vi "HMI.vi"() -> ()   [LabVIEW 2023]
uses:
  <vilib>/Instr/_visa.llb/VISA Configure Serial Port (Instr).vi
panel:
  out "reactiva":dbl
  out "aparente":dbl
  out "voltage":dbl
  out "corriente":dbl
  out "Fp":dbl
  in  "VISA resource name":refnum<visa-resource-name>
  out "Meter":dbl(knob) scale=0.001..1.0
  out "Voltaje (Señal control)":dynamicdata(graph)
  out "Numeric 3":dbl format="%#.2g"
  out "s? t:f 3":string
  out "s? t:f 2":string
  out "Numeric 2":dbl format="%#.2g"
  out "s? t:f":string
  out "Numeric":dbl format="%#.2g"
  in  "stop":bool
  out "1w 2":dbl(knob) scale=0.0..1.0
  out "10w 2":dbl(knob) scale=0.0..10.0
  out "100w":dbl(knob) scale=0.0..400.0
  out "10A 2":dbl(knob) scale=0.0..10.0
  out "1A":dbl(knob) scale=0.0..1.0
  out "1v":dbl(knob) scale=0.0..1.0
  out "10v":dbl(knob) scale=0.0..10.0
  out "100v":dbl(knob) scale=0.0..120.0
  # "ANALISIS ELECTRICO DEL SISTEMA ENERGETICO"
  # "Factor de Potencia"
  # "POTENCIA"
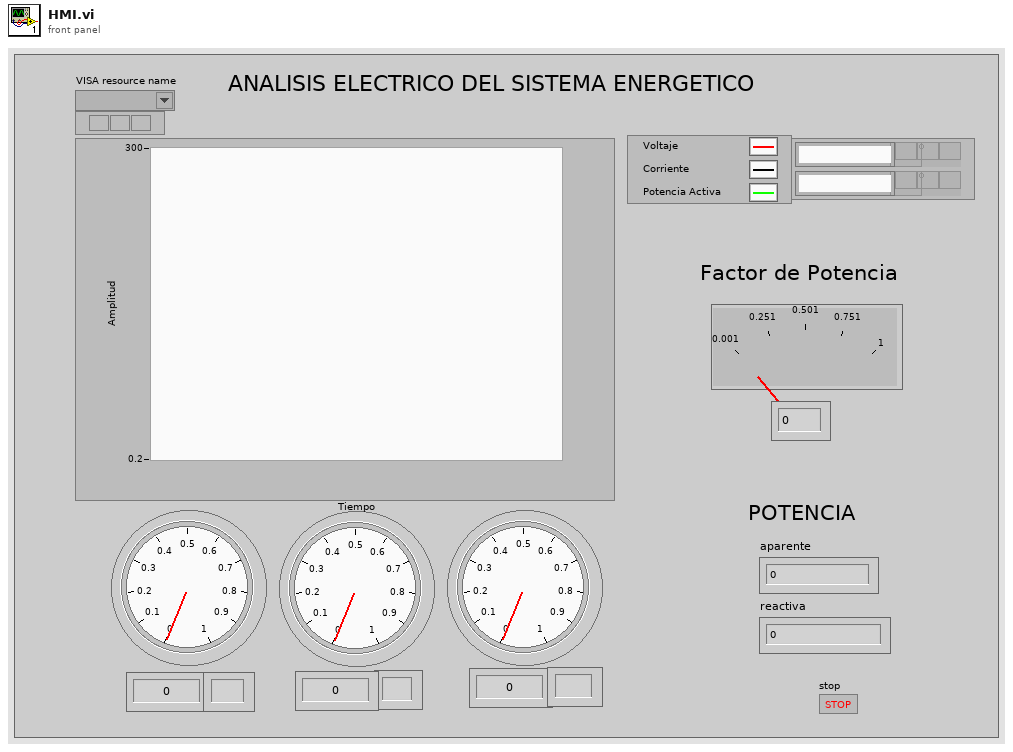
[diagram p1: front panel]
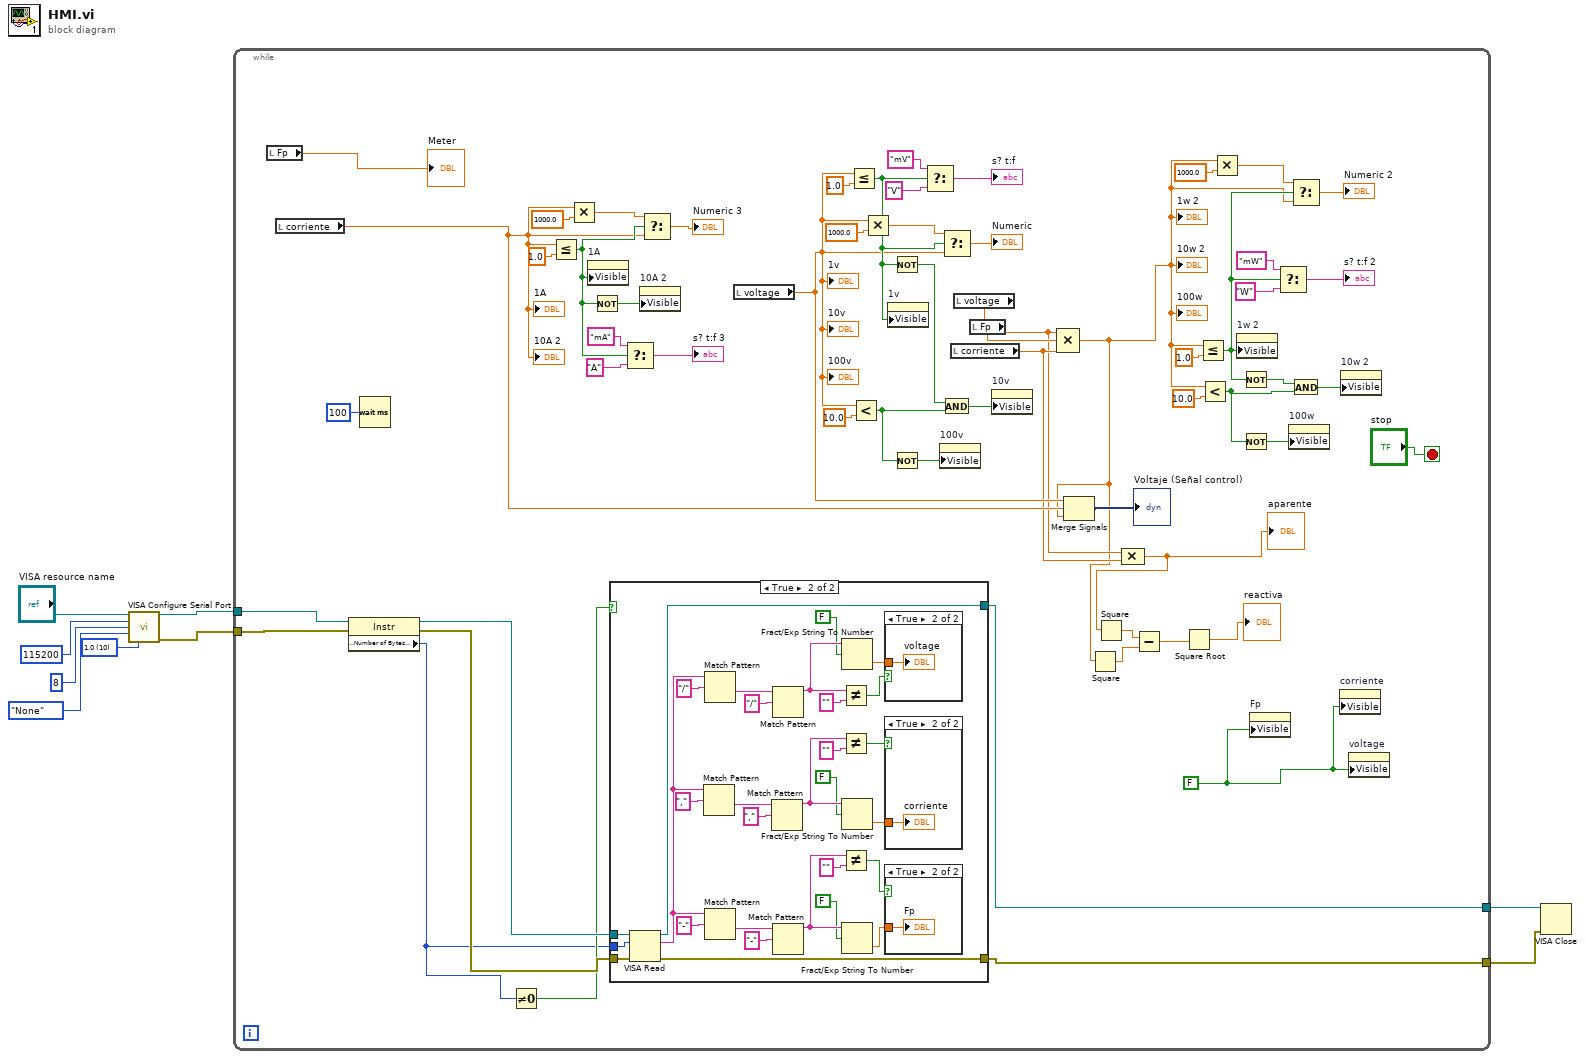
[diagram p0: block diagram]
diagram:
  w5 = u16 10 items=["1.0"=10, "1.5"=15, "2.0"=20] ("stop bits (10: 1 bit)")
  n1 = call-poly "VISA Configure Serial Port"("VISA resource name"="VISA resource name", "baud rate (9600)"=u32 115200, "data bits (8)"=u16 8, "parity (0:none)"=enum16{"None", "Odd", "Even", "Mark", "Space"}."None", "stop bits (10: 1 bit)"=w5) -> ("VISA resource name out"=w4:refnum<visa-resource-name>, "error out"=w3:errorcluster)  [unwired: 9 in]
  n2 = while {
    tunnel: w4 -> [w31]
    tunnel: w3 -> [w30]
    tunnel: [w26] -> w2
    tunnel: [w25] -> w1
    stop <- "stop" stop-if-true
    w22 = FALSE ("Visible")
    n3 = local read "Fp"() -> (→"Meter":dbl)
    n4 = local read "corriente"() -> (w20:dbl)
    "1A" <- w20
    "10A 2" <- w20
    n5 = property class="Instr"(reference=w31, error in=w30) -> (reference out=w28:refnum<visa-resource-name>, error out=w29:errorcluster, "Serial Settings:Number of Bytes at Serial Port"=w23:u32)
    n6 = Wait (ms)(milliseconds to wait=u32 100) -> ()  [unwired: 1 out]
    n7 = Not Equal To 0?(x=w23) -> (x != 0?=w24:bool)
    n8 = Less Or Equal?(x=w20, y=1.0) -> (x <= y?=w35:bool)
    n9 = Multiply(x=w20, y=1000.0) -> (x*y=w34:dbl)
    n10 = property on="1A" class="Knob (strict)"("Visible"=w35) -> ()  [unwired: 2 in, 2 out]
    n11 = Not(x=w35) -> (.not. x?=w38:bool)
    n12 = case shown="True" w24 {
      tunnel: [w69 w100] -> w25
      tunnel: [w70 w99] -> w26
      tunnel: w28 -> [w70 w98]
      tunnel: w29 -> [w69 w97]
      tunnel: w23 -> [_ w96]
      frame False {
      }
      frame True {
        n13 = VISA Read(VISA resource name=w98, byte count=w96, error in (no error)=w97) -> (VISA resource name out=w99:refnum<visa-resource-name>, read buffer=w86:string, error out=w100:errorcluster)  [unwired: 1 out]
        n14 = Match Pattern(string=w86, regular expression=",") -> (after substring=w93:string)  [unwired: 1 in, 3 out]
        n15 = Match Pattern(string=w86, regular expression="/") -> (after substring=w87:string)  [unwired: 1 in, 3 out]
        n16 = Match Pattern(string=w86, regular expression="-") -> (after substring=w90:string)  [unwired: 1 in, 3 out]
        n17 = Match Pattern(string=w93, regular expression=",") -> (before substring=w75:string)  [unwired: 1 in, 3 out]
        n18 = Match Pattern(string=w87, regular expression="/") -> (before substring=w84:string)  [unwired: 1 in, 3 out]
        n19 = Match Pattern(string=w90, regular expression="-") -> (before substring=w74:string)  [unwired: 1 in, 3 out]
        n20 = Not Equal?(x=w84, y="") -> (x != y?=w77:bool)
        n21 = Not Equal?(x=w75, y="") -> (x != y?=w79:bool)
        n22 = Not Equal?(x=w74, y="") -> (x != y?=w80:bool)
        n23 = Fract/Exp String To Number(use system decimal point (T)=FALSE, string=w84) -> (number=w76:dbl)  [unwired: 2 in, 1 out]
        n24 = Fract/Exp String To Number(use system decimal point (T)=FALSE, string=w75) -> (number=w78:dbl)  [unwired: 2 in, 1 out]
        n25 = Fract/Exp String To Number(use system decimal point (T)=FALSE, string=w74) -> (number=w81:dbl)  [unwired: 2 in, 1 out]
        n26 = case shown="True" w77 {
          tunnel: w76 -> [_ w103]
          frame False {
          }
          frame True {
            "voltage" <- w103
          }
        }
        n27 = case shown="True" w79 {
          tunnel: w78 -> [_ w102]
          frame False {
          }
          frame True {
            "corriente" <- w102
          }
        }
        n28 = case shown="True" w80 {
          tunnel: w81 -> [_ w101]
          frame False {
          }
          frame True {
            "Fp" <- w101
          }
        }
      }
    }
    n29 = Select(t="mA", s=w35, f="A") -> (s? t:f=→"s? t:f 3":string)
    n30 = property on="10A 2" class="Knob (strict)"("Visible"=w38) -> ()  [unwired: 2 in, 2 out]
    n31 = Select(t=w34, s=w35, f=w20) -> (s? t:f=→"Numeric 3":dbl)
    n32 = local read "voltage"() -> (w19:dbl)
    "100v" <- w19
    "10v" <- w19
    "1v" <- w19
    n33 = Less Or Equal?(x=w19, y=1.0) -> (x <= y?=w52:bool)
    n34 = Less?(x=w19, y=10.0) -> (x < y?=w60:bool)
    n35 = Multiply(x=w19, y=1000.0) -> (x*y=w53:dbl)
    n36 = property on="1v" class="Knob (strict)"("Visible"=w52) -> ()  [unwired: 2 in, 2 out]
    n37 = Not(x=w52) -> (.not. x?=w61:bool)
    n38 = Not(x=w60) -> (.not. x?=w55:bool)
    n39 = Select(t="mV", s=w52, f="V") -> (s? t:f=→"s? t:f":string)
    n40 = property on="100v" class="Knob (strict)"("Visible"=w55) -> ()  [unwired: 2 in, 2 out]
    n41 = Select(t=w53, s=w52, f=w19) -> (s? t:f=→"Numeric":dbl)
    n42 = And(x=w61, y=w60) -> (x .and. y?=w57:bool)
    n43 = local read "corriente"() -> (w17:dbl)
    n44 = local read "voltage"() -> (w16:dbl)
    n45 = local read "Fp"() -> (w18:dbl)
    n46 = property on="10v" class="Knob (strict)"("Visible"=w57) -> ()  [unwired: 2 in, 2 out]
    n47 = Compound Arithmetic op=MULTIPLY(w16, w18, w17) -> (w11:dbl)
    "100w" <- w11
    "10w 2" <- w11
    "1w 2" <- w11
    n48 = Merge Signals(w19, w20, w11) -> (→"Voltaje (Señal control)":dynamicdata)
    n49 = Square(x=w11) -> (x^2=w14:dbl)
    n50 = Compound Arithmetic op=MULTIPLY(w16, w17) -> (w12:dbl)
    "aparente" <- w12
    n51 = Square(x=w12) -> (x^2=w13:dbl)
    n52 = Subtract(x=w13, y=w14) -> (x-y=w15:dbl)
    n53 = Square Root(x=w15) -> (sqrt(x)=→"reactiva":dbl)
    n54 = Less Or Equal?(x=w11, y=1.0) -> (x <= y?=w42:bool)
    n55 = Less?(x=w11, y=10.0) -> (x < y?=w64:bool)
    n56 = Multiply(x=w11, y=1000.0) -> (x*y=w46:dbl)
    n57 = property on="1w 2" class="Knob (strict)"("Visible"=w42) -> ()  [unwired: 2 in, 2 out]
    n58 = Not(x=w42) -> (.not. x?=w65:bool)
    n59 = Not(x=w64) -> (.not. x?=w59:bool)
    n60 = property on="Fp" class="DigNum (strict)"("Visible"=w22) -> ()  [unwired: 2 in, 2 out]
    n61 = Select(t="mW", s=w42, f="W") -> (s? t:f=→"s? t:f 2":string)
    n62 = property on="100w" class="Knob (strict)"("Visible"=w59) -> ()  [unwired: 2 in, 2 out]
    n63 = Select(t=w46, s=w42, f=w11) -> (s? t:f=→"Numeric 2":dbl)
    n64 = And(x=w65, y=w64) -> (x .and. y?=w58:bool)
    n65 = property on="corriente" class="DigNum (strict)"("Visible"=w22) -> ()  [unwired: 2 in, 2 out]
    n66 = property on="10w 2" class="Knob (strict)"("Visible"=w58) -> ()  [unwired: 2 in, 2 out]
    n67 = property on="voltage" class="DigNum (strict)"("Visible"=w22) -> ()  [unwired: 2 in, 2 out]
  }
  n68 = VISA Close(VISA resource name=w2, error in (no error)=w1) -> ()  [unwired: 1 out]
